vi "transfer char run_subvi_14_2014 05 29_JWc.vi"(0 "VISA session":refnum<visa-resource-name>="GPIB0::17::INSTR", 1 "Y2 axis settings":T7={"Y2 axis on/off"=FALSE, "MINIMUM"=0.0, "MAXIMUM"=1.0, "Variable name"="Ig", "LIN or LOG axis"="LIN"} {"MAXIMUM" format="%.9f"; "MINIMUM" format="%.9f"}, 3 "LKG Path":path, 5 "Var1 sweep settings":T9={"start"=40.0, "stop"=-40.0, "step (linear only)"=-1.0, "sweep spacing (linear: 0)"=0, "sweep mode"=FALSE, "compliance (V)"=100.0, "compliance (A)"=0.001} {"compliance (A)" format="%^.2e"; "compliance (V)" format="%.2f"; "sweep spacing (linear: 0)" items=["linear", "log 10", "log 25", "log 50"]; "step (linear only)" format="%.2f"; "stop" format="%.2f"; "start" format="%.2f"}, 7 "Var2 step settings":T8={"compliance (A)"=0.001, "compliance (V)"=100.0, "start"=-2.0, "total points"=2, "step"=-38.0} {"step" format="%.2f"; "start" format="%.2f"; "compliance (V)" format="%.2f"; "compliance (A)" format="%^.2e"}, 9 "integration time":u32(slide) scale=0.0..2.0, 11 "Input Path":path, 12 "Dielectric Constant":dbl=5.0, 13 "Sample Properties:":T6 {"Date Created" format="%<%x>T"}) -> (2 "Check Cluster":T4, 4 "Output":T5 {"Mobility-Lin" format="%#_4e"; "Mobility-Sat" format="%#_4e"}, 6 "Graph Cluster":T3, 15 "Error In":errorcluster)   [LabVIEW 2012]
panel:
  in  "Y1 Axis Settings":T1={"Y1 axis"="Id", "MINIMUM"=-1e-05, "MAXIMUM"=0.0, "LIN or LOG axis"="LIN"} {"MAXIMUM" format="%.2e"; "MINIMUM" format="%_2e"}
  in  "SMU Config":T2={"Vname"="Vs", "Vname 2"="Vd", "Vname 3"="Vg", "Vname 4"="V4", "Iname"="Is", "Iname 2"="Id", "Iname 3"="Ig", "Iname 4"="I4", "Mode"=4, "Mode 2"=0, "Mode 3"=0, "Mode 4"=0, "Function"=4, "Function 2"=2, "Function 3"=1, "Function 4"=4, "Value (V or A)"=0.0, "Value (Either V or A) 2"=0.0, "Value (Either V or A) 3"=0.0, "Value (Either V or A) 4"=0.0} {"Function" items=["disabled", "Var1", "Var2", "Var1'", "Constant"]; "Mode" items=["V", "I", "VPulse", "IPulse", "Common"]; "Function 4" items=["disabled", "Var1", "Var2", "Var1'", "Constant"]; "Mode 4" items=["V", "I", "VPulse", "IPulse", "Common"]; "Function 3" items=["disabled", "Var1", "Var2", "Var1'", "Constant"]; "Mode 3" items=["V", "I", "VPulse", "IPulse", "Common"]; "Function 2" items=["disabled", "Var1", "Var2", "Var1'", "Constant"]; "Mode 2" items=["V", "I", "VPulse", "IPulse", "Common"]}
  in  "Output Path":path
  in  "Temp (K)":dbl=0.001 format="%^.2e"
  in  "NumPts":dbl=5.0
  out "Error Out":errorcluster
  out "Gate Current Plot":cluster{"trace":dbl[], "trace":dbl[]}(graph)
  out "graphic display":cluster{"trace":dbl[], "trace":dbl[]}(graph)
  in  "wait time parameter":dbl=1.0
  in  "compliance (A)":dbl=0.001 format="%^.2e"
  in  "compliance (V)":dbl=100.0 format="%^.2e"
  in  "reset":bool=TRUE
  # "SMU1"
  # "SMU2"
  # "SMU3"
  # "SMU4"
  # "Sample Properties:"
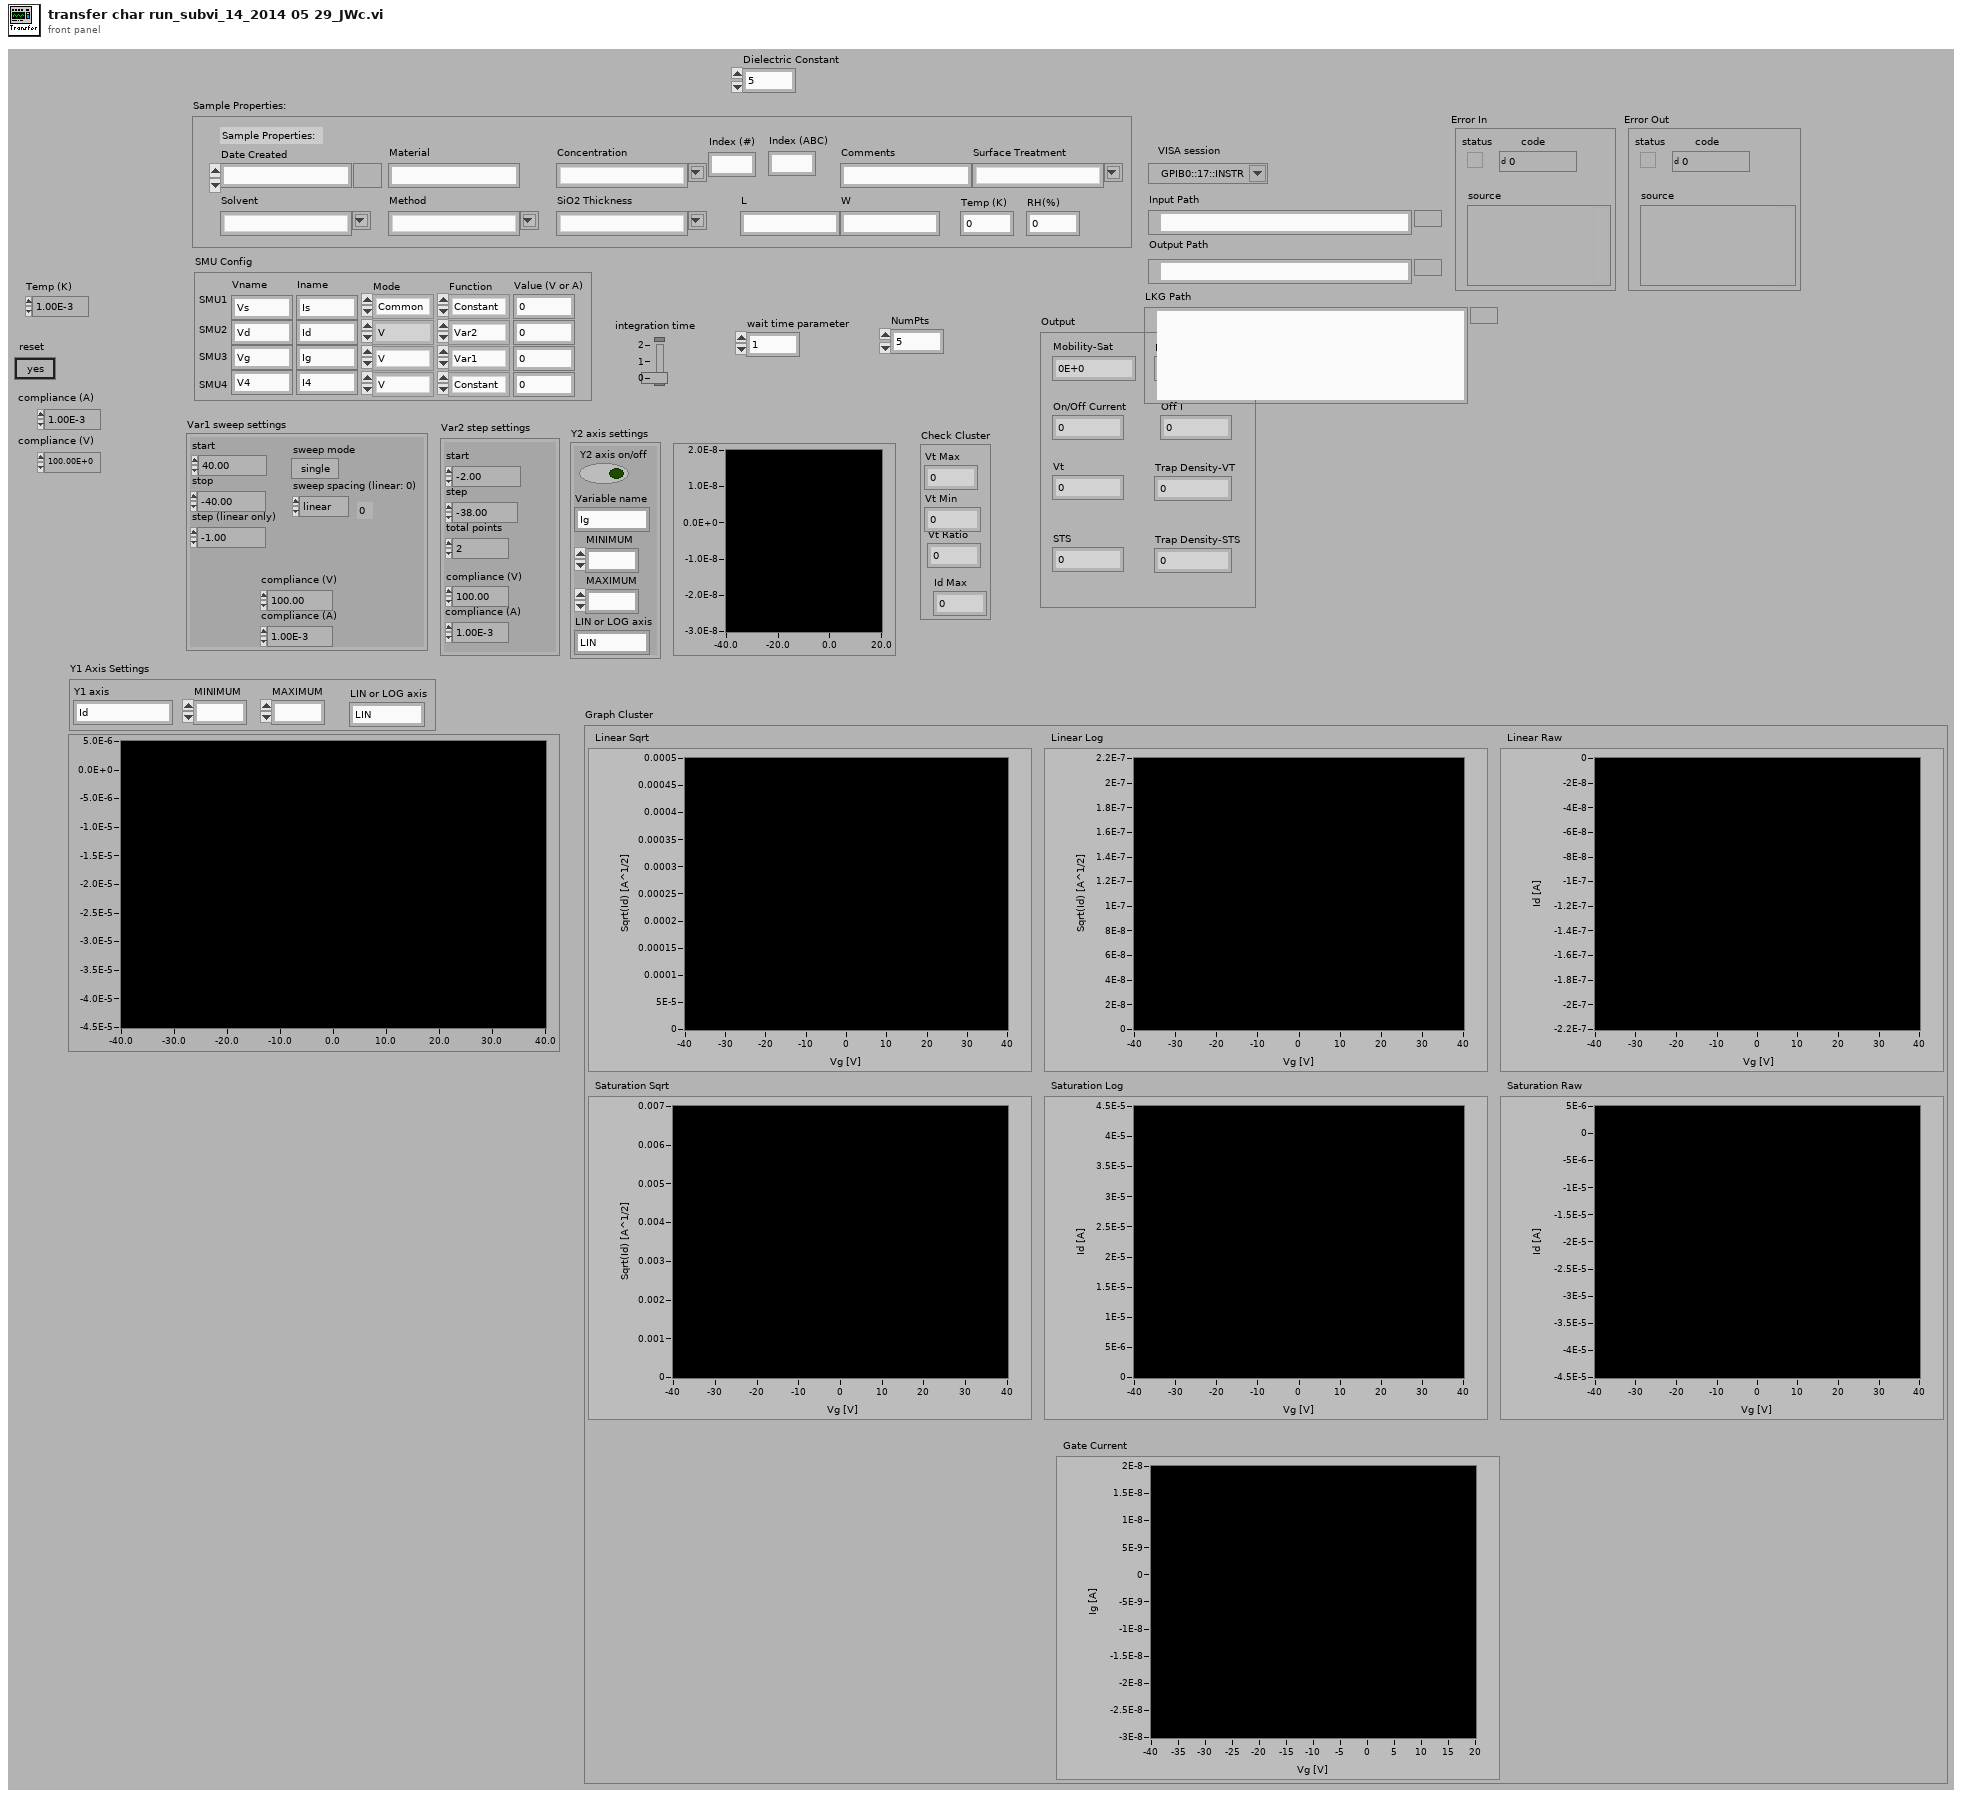
[diagram p1: front panel]
types:
  T1 = cluster{"Y1 axis":string, "MINIMUM":ext, "MAXIMUM":ext, "LIN or LOG axis":string}
  T2 = cluster{"Vname":string, "Vname 2":string, "Vname 3":string, "Vname 4":string, "Iname":string, "Iname 2":string, "Iname 3":string, "Iname 4":string, "Mode":u16, "Mode 2":u16, "Mode 3":u16, "Mode 4":u16, "Function":u16, "Function 2":u16, "Function 3":u16, "Function 4":u16, "Value (V or A)":dbl, "Value (Either V or A) 2":dbl, "Value (Either V or A) 3":dbl, "Value (Either V or A) 4":dbl}
  T3 = cluster{"Linear Sqrt":cluster{dbl[], "trace":dbl[]}[], "Linear Log":cluster{dbl[], "trace":dbl[]}[], "Linear Raw":cluster{dbl[], dbl[]}[], "Saturation Sqrt":cluster{dbl[], "trace":dbl[]}[], "Saturation Log":cluster{dbl[], "trace":dbl[]}[], "Saturation Raw":cluster{dbl[], "trace":dbl[]}[], "Gate Current":cluster{dbl[], "trace":dbl[]}[]}
  T4 = cluster{"Vt Max":i32, "Vt Min":i32, "Vt Ratio":i32, "Id Max":dbl}
  T5 = cluster{"Mobility-Sat":dbl, "Mobility-Lin":dbl, "On/Off Current":dbl, "Off I":dbl, "Vt":dbl, "STS":dbl, "Trap Density-VT":dbl, "Trap Density-STS":dbl}
  T6 = cluster{"Date Created":timestamp, "Material":string, "Solvent":string, "Concentration":string, "Method":string, "SiO2 Thickness":string, "Index (#)":string, "Index (ABC)":string, "L":string, "W":string, "Surface Treatment":string, "Comments":string, "Temp (K)":dbl, "RH(%)":dbl}
  T7 = cluster{"Y2 axis on/off":bool, "MINIMUM":ext, "MAXIMUM":ext, "Variable name":string, "LIN or LOG axis":string}
  T8 = cluster{"compliance (A)":dbl, "compliance (V)":dbl, "start":dbl, "total points":u16, "step":dbl}
  T9 = cluster{"start":dbl, "stop":dbl, "step (linear only)":dbl, "sweep spacing (linear: 0)":u16, "sweep mode":bool, "compliance (V)":dbl, "compliance (A)":dbl}
  T10 = cluster{"spreadsheet string":string, "spreadsheet string":string, "spreadsheet string":string}
  T11 = cluster{"Mobility-Sat":dbl, "Mobility-Lin":dbl, "On/Off I-Sat":dbl, "Off I-Sat":dbl, "VT-Sat":dbl, "Sub Threshold Swing":dbl, "Trap Density-VT":dbl, "Trap Density (N)":dbl}
  T12 = cluster{"Vt Max":dbl, "Vt Min":dbl, "Vt Ratio":dbl, "Id Max":dbl}
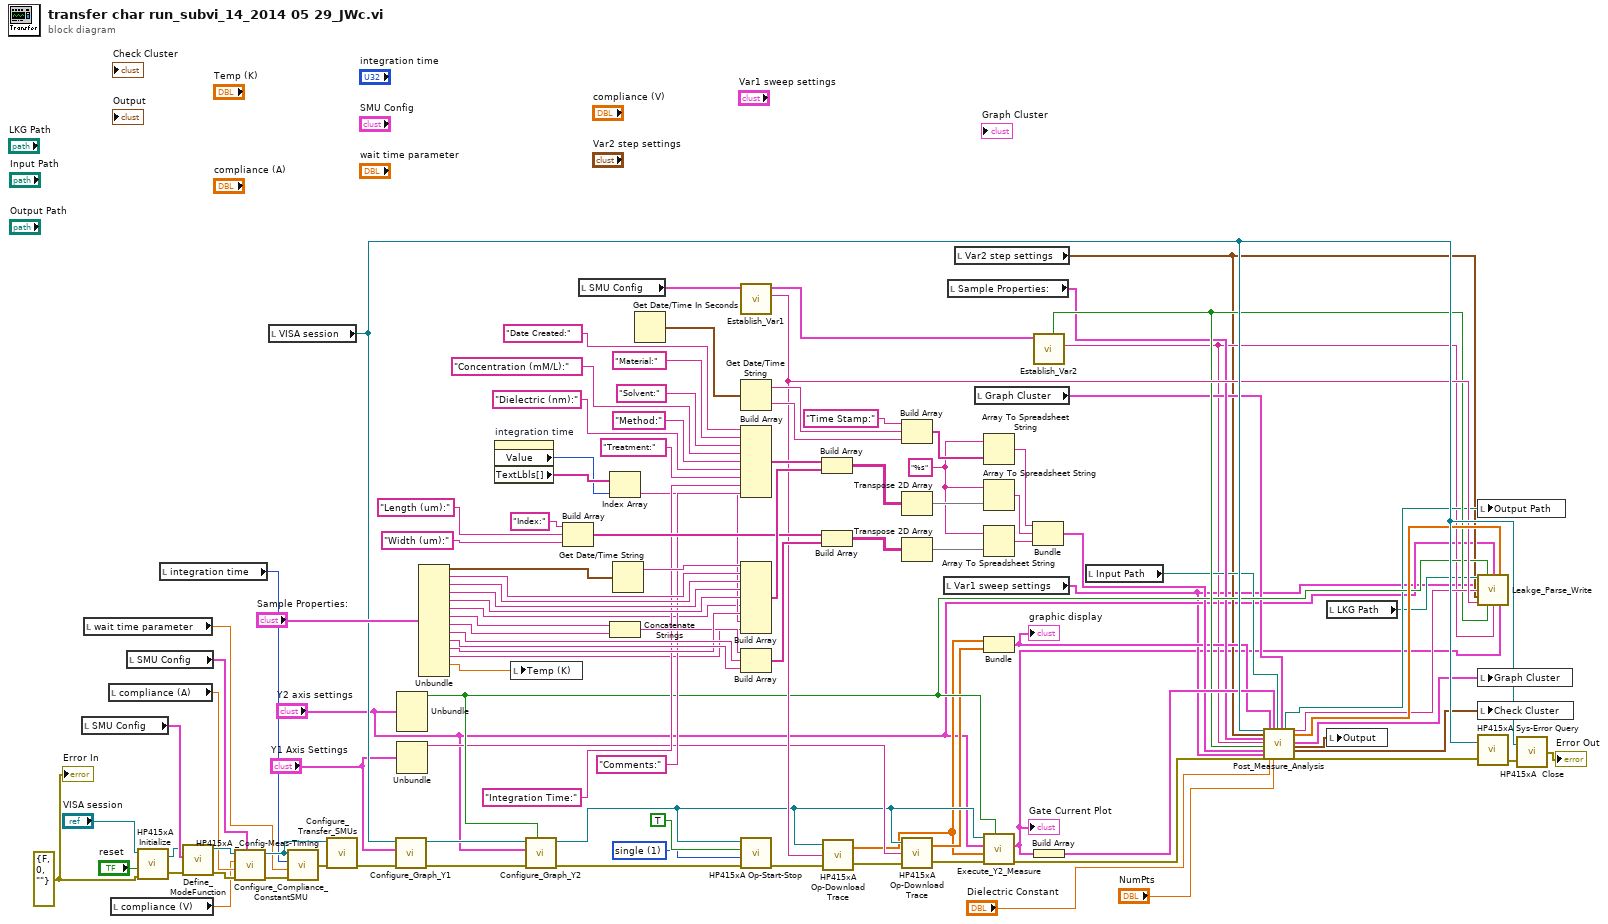
[diagram p0: block diagram]
diagram:
  w39 = u32 1 items=["stop  ", "single  ", "single-append  ", "stress start  ", "continuous  ", "standby on  ", "standby off  ", "zero  "] ("function (stop:0)")
  w45 = errorcluster {"status"=FALSE, "code"=0, "source"=""} ("error out")
  w68 = "%s"
  n1 = local read "SMU Config"() -> (w50:T2)
  n2 = local read "wait time parameter"() -> (w53:dbl)
  n3 = local read "compliance (A)"() -> (w49:dbl)
  n4 = local read "compliance (V)"() -> (w48:dbl)
  n5 = local read "SMU Config"() -> (w51:T2)
  n6 = call "HP415xA  Initialize.vi"("instrument descriptor"="VISA session", "reset"="reset", "error in (no error)"=w45) -> ("VISA session"=w47:refnum<visa-resource-name>, "error out"=w55:errorcluster)  [unwired: 2 in]
  n7 = local read "integration time"() -> (w54:u32)
  n8 = call "Define_ModeFunction.vi"("error in (no error)"=w55, "SMU Config"=w50, "VISA Refnum in"=w47) -> ("error out"=w56:errorcluster, "VISA Refnum out"=w58:refnum<visa-resource-name>)  [unwired: 7 in]
  n9 = call "Configure_Compliance_ConstantSMU.vi"("SMU Config"=w51, "error in (no error)"=w56, "compliance (A)"=w49, "compliance (V)"=w48, "VISA In"=w58) -> ("error out"=w57:errorcluster, "VISA Out"=w59:refnum<visa-resource-name>)  [unwired: 5 in]
  n10 = local read "VISA session"() -> (w60:refnum<visa-resource-name>)
  n11 = call "HP415xA _Config-Meas-Timing.vi"("error in (no error)"=w57, "wait time parameter"=w53, "integration time"=w54, "VISA session"=w59) -> ("error out"=w52:errorcluster)  [unwired: 2 in]
  n12 = call "Configure_Transfer_SMUs.vi"("error in (no error)"=w52, "VISA In"=w59) -> ("error out"=w3:errorcluster)  [unwired: 8 in, 1 out]
  n13 = call "Configure_Graph_Y1.vi"("error in (no error)"=w3, "Y1 Axis Settings"="Y1 Axis Settings", "VISA In"=w60) -> ("error out"=w36:errorcluster, "VISA Out"=w23:refnum<visa-resource-name>)  [unwired: 7 in]
  n14 = Unbundle("Y2 axis settings") -> ("Y2 axis on/off"=w26:bool)  [unwired: 4 out]
  n15 = Unbundle("Y1 Axis Settings") -> ("Y1 axis"=w25:string)  [unwired: 3 out]
  n16 = Unbundle("Sample Properties:") -> ("Date Created"=w81:timestamp, "Material"=w80:string, "Solvent"=w77:string, "Concentration"=w76:string, "Method"=w79:string, "SiO2 Thickness"=w43:string, "Index (#)"=w72:string, "Index (ABC)"=w71:string, "L"=w74:string, "W"=w75:string, "Surface Treatment"=w73:string, "Comments"=w65:string, "Temp (K)"=w69:dbl)  [unwired: 1 out]
  n17 = property on="integration time" class="Slide (strict)"() -> ("Value"=w63:u32, "TextLbls[]"=w64:string[])  [unwired: 2 in, 2 out]
  n18 = local write "Temp (K)"(w69) -> ()
  n19 = call "Configure_Graph_Y2.vi"("Execute?"=w26, "error in (no error)"=w36, "Y2 axis settings"="Y2 axis settings", "VISA In"=w23) -> ("error out"=w37:errorcluster, "VISA Out"=w22:refnum<visa-resource-name>)  [unwired: 6 in]
  n20 = Build Array("Index:", "Length (um):", "Width (um):") -> (w87:string[])
  n21 = local read "SMU Config"() -> (w61:T2)
  n22 = Index Array(array=w64, index=w63) -> (element=w62:string)
  n23 = Concatenate Strings(w72, w71) -> (w70:string)
  n24 = Get Date/Time String(seconds (now)=w81) -> (date string=w107:string)  [unwired: 2 in, 1 out]
  n25 = Get Date/Time In Seconds() -> (seconds since 1Jan1904=w102:timestamp)
  n26 = call "Establish_Var1.vi"("SMU Config In"=w61) -> ("Vname"=w30:string, "SMU Config Out"=w27:T2)  [unwired: 8 in]
  n27 = Get Date/Time String(seconds (now)=w102) -> (date string=w101:string, time string=w100:string)  [unwired: 2 in]
  n28 = Build Array("Date Created:", "Material:", "Solvent:", "Concentration (mM/L):", "Method:", "Dielectric (nm):", "Treatment:", "Integration Time:", "Comments:") -> (w91:string[])
  n29 = Build Array(w107, w80, w77, w76, w79, w43, w73, w62, w65) -> (w90:string[])
  n30 = Build Array(w70, w74, w75) -> (w86:string[])
  n31 = call "HP415xA Op-Start-Stop.vi"("error in (no error)"=w37, "function (stop:0)"=w39, "wait until finish"=TRUE, "VISA session"=w22) -> ("error out"=w38:errorcluster)  [unwired: 6 in, 1 out]
  n32 = Build Array(w91, w90) -> (w89:string[][])
  n33 = Build Array(w87, w86) -> (w85:string[][])
  n34 = call "HP415xA Op-Download Trace.vi"("error in (no error)"=w38, "trace (variable) name"=w30, "VISA session"=w22) -> ("error out"=w42:errorcluster, "trace"=w17:dbl[])
  n35 = Build Array("Time Stamp:", w101, w100) -> (w99:string[])
  n36 = Transpose 2D Array(2D array=w89) -> (transposed array=w88:string[][])
  n37 = Transpose 2D Array(2D array=w85) -> (transposed array=w84:string[][])
  n38 = call "HP415xA Op-Download Trace.vi"("error in (no error)"=w42, "trace (variable) name"=w25, "VISA session"=w22) -> ("error out"=w35:errorcluster, "trace"=w19:dbl[])
  n39 = local read "Var1 sweep settings"() -> (w5:T9)
  n40 = local read "Sample Properties:"() -> (w20:T6)
  n41 = local read "Var2 step settings"() -> (w7:T8)
  n42 = local read "Graph Cluster"() -> (w10:T3)
  n43 = Array To Spreadsheet String(array=w99, 3:w68) -> (spreadsheet string=w92:string)  [unwired: 1 in]
  n44 = Array To Spreadsheet String(array=w88, 3:w68) -> (spreadsheet string=w95:string)  [unwired: 1 in]
  n45 = Array To Spreadsheet String(array=w84, 3:w68) -> (spreadsheet string=w83:string)  [unwired: 1 in]
  n46 = Bundle("trace"=w17, "trace"=w19) -> (w18:cluster{"trace":dbl[], "trace":dbl[]})  [unwired: 1 in]
  "graphic display" <- w18
  n47 = call "Execute_Y2_Measure.vi"("VISA In"=w22, "Y2 axis settings"="Y2 axis settings", "X-Axis Trace"=w17, "error in (no error)"=w35, "Y2 axis on/off"=w26) -> ("Y2 Output Cluster"=w4:cluster{"trace":dbl[], "trace":dbl[]}, "error out"=w32:errorcluster)  [unwired: 4 in]
  "Gate Current Plot" <- w4
  n48 = Bundle("spreadsheet string"=w92, "spreadsheet string"=w95, "spreadsheet string"=w83) -> (w21:T10)  [unwired: 1 in]
  n49 = call "Establish_Var2.vi"("SMU Config In"=w27) -> ("Vname"=w9:string, "Execute?"=w28:bool)  [unwired: 8 in, 1 out]
  n50 = Build Array(w4) -> (w31:cluster{"trace":dbl[], "trace":dbl[]}[])
  n51 = local read "Input Path"() -> (w11:path)
  n52 = call "Post_Measure_Analysis.vi"("VISA Refnum in"=w60, "Var2 step settings"=w7, "Sample Properties:"=w20, "Vname"=w9, "Execute?"=w28, "Header Strings"=w21, "Var1 sweep settings"=w5, "error in (no error)"=w32, "Id Vg Data"=w18, "Dielectric Constant"="Dielectric Constant", "Gate Current"=w31, "NumPts"="NumPts", "Input Path"=w11, "Graph Cluster in"=w10) -> ("File out"=w12:path, "Header out"=w29:string, "Vd Data"=w33:dbl[], "Graph Cluster out"=w16:T3, "Device Properties Out"=w15:T11, "Check Cluster"=w14:T12, "error out"=w34:errorcluster)  [unwired: 5 in, 2 out]
  n53 = local read "LKG Path"() -> (w8:path)
  n54 = local write "Output"(w15) -> ()
  n55 = local write "Output Path"(w12) -> ()
  n56 = call "Leakge_Parse_Write.vi"("LKG Path"=w8, "Y2 axis on/off"=w26, "Y2 axis settings"="Y2 axis settings", "Vd Data"=w33, "Var1 sweep settings"=w5, "Header in"=w29, "Var2 step settings"=w7, "Vname 2"=w30, "Execute?"=w28, "Vname"=w9, "Y2 Output Cluster"=w4) -> ()  [unwired: 5 in]
  n57 = local write "Graph Cluster"(w16) -> ()
  n58 = local write "Check Cluster"(w14) -> ()
  n59 = call "HP415xA Sys-Error Query.vi"("VISA session"=w60, "error in (no error)"=w34) -> ("error out"=w41:errorcluster)  [unwired: 2 in, 1 out]
  n60 = call "HP415xA  Close.vi"("error in (no error)"=w41, "VISA session"=w60) -> ("error out"=→"Error Out":errorcluster)
  "Error In" <- w45
